vi "dfd_MA_Decimation Filter.vi"(0 "input data":fxp<+/-,16,16>, 9 "input valid":bool=TRUE) -> (4 "output data":fxp<+/-,32,32>, 10 "output valid":bool, 14 "ready for input":bool)   [LabVIEW 2017]
uses:
  <vilib>/rvi/FXPMathLib/basic elements/FxpIntAccumulator/subVIs/nifxpmath_IntAccumulator_SimConfig.ctl
  <vilib>/rvi/FXPMathLib/basic elements/FxpIntAccumulator/simVIs/DllFxpIntAccumulator_sub.vi
  <vilib>/rvi/FXPMathLib/basic elements/FxpIntAccumulator/XNode/nifxpmath_IntAccumulator.xnode
  <vilib>/rvi/FXPMathLib/FxpMul/XNode/nifxpmath_Multiplier.xnode
  <vilib>/rvi/FXPMathLib/basic elements/FxpDiscreteDelay/XNode/nifxpmath_DiscreteDelay.xnode
  <vilib>/rvi/FXPMathLib/basic elements/FxpAddSub/XNode/nifxpmath_AddSub.xnode
  <vilib>/rvi/FXPMathLib/sim/FxpSim.dll
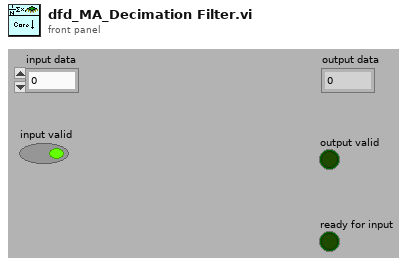
[diagram p1: front panel]
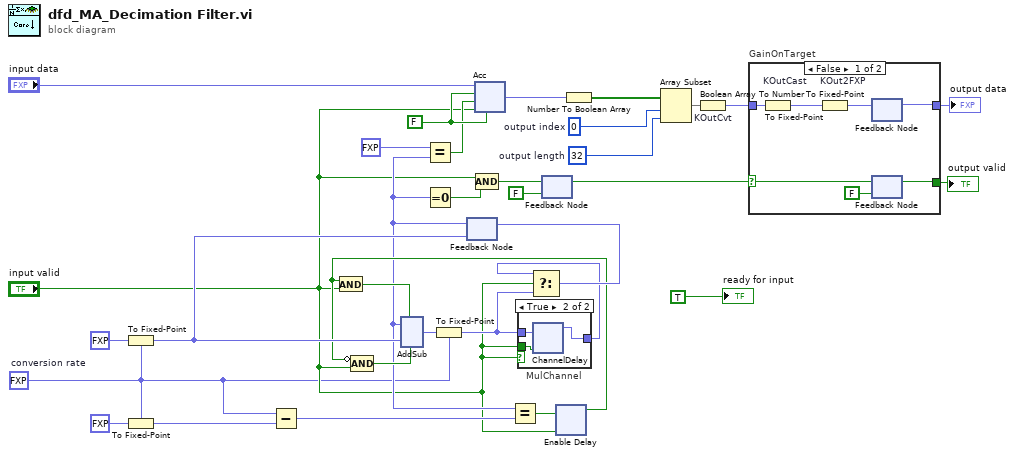
[diagram p0: block diagram]
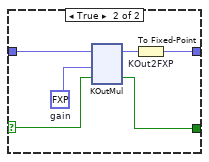
[diagram p2: hidden frame]
diagram:
  w1 = fxp<+,2,2> 3.0  # conversion rate
  w10 = 32  # output length
  w11 = 0  # output index
  w18 = FALSE ("carry-in/no borrow-in")
  n1 = To Fixed-Point(fixed-point type=w1, number=fxp<+,2,2> 0.0 ("fixed-point")) -> (fixed-point=w33:fxp<+,2,2>)
  n2 = To Fixed-Point(fixed-point type=w1, number=fxp<+,2,2> 2.0 ("fixed-point")) -> (fixed-point=w32:fxp<+,2,2>)
  n3 = Subtract(x=w1, y=w32) -> (x-y=w31:fxp<+/-,3,3>)
  n4 = feedback #1(w33) -> (w14:fxp<+,2,2>)
  n5 = Equal?(x=fxp<+,1,1> 1.0, y=w14) -> (x = y?=w16:bool)
  n6 = Equal To 0?(x=w14) -> (x = 0?=w29:bool)
  n7 = xnode "Acc"("x"="input data", "load (F)"=w16, "is sub? (F)"=w18, "enable (T)"="input valid", "carry-in/inverted borrow-in (F)"=w18) -> ("s"=w8:fxp<+/-,48,48>)  [unwired: 1 out]
  n8 = Compound Arithmetic op=AND("input valid", w29) -> (w21:bool)
  n9 = Equal?(x=w14, y=w31) -> (x = y?=w23:bool)
  n10 = feedback-in #2(w21) -> ()
  n11 = feedback #2(FALSE) -> (w6:bool)
  n12 = xnode "Enable Delay"("D"=w23, "enable"="input valid") -> ("Q"=w22:bool)
  n13 = And(x=w22, y="input valid") -> (x .and. y?=w26:bool)
  n14 = Compound Arithmetic op=AND(invert w22, "input valid") -> (w30:bool)
  n15 = xnode ("AddSub")("x"=w14, "y"=w33, "carry-in"=w30, "use zero instead of x"=w26) -> ("s"=w25:fxp<+,2,2>)  [unwired: 1 out]
  n16 = To Fixed-Point(fixed-point type=w1, number=w25) -> (fixed-point=w24:fxp<+,2,2>)
  n17 = case "MulChannel" shown="True" "input valid" {
    tunnel: [w34 w37] -> w27
    tunnel: w24 -> [w34 w36]
    tunnel: "input valid" -> [_ w35]
    frame False {
    }
    frame True {
      n18 = xnode ("ChannelDelay")("D"=w36, "enable"=w35) -> ("Q"=w37:fxp<+,2,2>)
    }
  }
  n19 = Select(t=w27, s="input valid", f=w24) -> (s? t:f=w28:fxp<+,2,2>)
  n20 = feedback-in #1(w28) -> ()
  n21 = Number To Boolean Array(number=w8) -> (Boolean array=w7:bool[])
  n22 = Array Subset(array=w7, index=w11, length=w10) -> (w9:bool[])
  n23 = Boolean Array To Number "KOutCvt"(Boolean array=w9) -> (number=w12:fxp<+/-,32,32>)
  n24 = case "GainOnTarget" shown="False" w6 {
    selector: w6 -> [w40 w46]
    tunnel: [w42 w50] -> w5
    tunnel: [w43 w48] -> w4
    tunnel: w12 -> [w39 w47]
    frame False {
      n25 = To Fixed-Point "KOutCast"(number=w39) -> (fixed-point=w38:fxp<+/-,32,32>)  [unwired: 1 out]
      n26 = To Fixed-Point "KOut2FXP"(number=w38) -> (fixed-point=w41:fxp<+/-,32,32>)  [unwired: 1 out]
      n27 = feedback-in #3(w41) -> ()
      n28 = feedback #3() -> (w43:fxp<+/-,32,32>)  [unwired: 1 out]
      n29 = feedback-in #4(w40) -> ()
      n30 = feedback #4(FALSE ("input valid")) -> (w42:bool)
    }
    frame True {
      w49 = fxp<+/-,16,1> 0.0  # gain
      n31 = xnode "KOutMul"("x"=w47, "y"=w49, "input valid"=w46) -> ("x*y"=w45:fxp<+/-,32,32>, "output valid"=w50:bool)  [unwired: 1 in, 1 out]
      n32 = To Fixed-Point "KOut2FXP"(number=w45) -> (fixed-point=w48:fxp<+/-,32,32>)  [unwired: 1 out]
    }
  }
  "output valid" <- w5
  "output data" <- w4
  "ready for input" <- TRUE
